vi "Mouse Down.vi"(8 "error in":errorcluster, 10 "Double Click":bool, 11 "Data in":T1={"Class"={"Ants"=refnum, "Layer"=refnum, "Templates"=refnum, "Icon"=refnum, "Glyph"=refnum, "Settings"=refnum, "Tools"=refnum, "History"=refnum}, "Ref"={"Add Layer"=refnum, "Remove Layer"=refnum, "Line Text"=[], "Body Text Spec"=refnum, "DNL_Font"=refnum, "glyph path str"=refnum, "templates path str"=refnum, "Arrow Up"=refnum, "Arrow Down"=refnum, "IE VI Ref"=refnum, "Glyphs tree"=refnum, "Templates tree"=refnum, "Layer Icon Text"=refnum, "Layer Template"=refnum, "Body Text"=refnum, "Search Templates"=refnum, "TextMarker"=refnum, "Tab Control"=refnum, "Search Glyphs"=refnum, "Line Color"=refnum, "DNL_Glyphs []"=refnum, "Fill Color"=refnum, "Tools"=refnum, "Icon"=refnum, "Preview"=refnum, "Ants"=refnum, "Terminals"=refnum, "menu reference"=refnum, "LayerNames"=[], "GlyphLoadAnimation"=refnum, "TemplateLoadAnimation"=refnum, "refreshGlyphs"=refnum, "refreshTemplates"=refnum}, "Support"={"AntsRect"={"left"=0, "top"=0, "right"=0, "bottom"=0}, "Mouse Move Coords"={"Horizontal"=0, "Vertical"=0}, "Mouse Down Coords"={"Horizontal"=0, "Vertical"=0}, "Temp Coord"={"Horizontal"=0, "Vertical"=0}, "Action"=enum."Default", "Edge Color"=4914962, "Fill Color"=16860, "Mouse Down?"=FALSE, "Draft Mode?"=FALSE, "Temp Icon"=bytes[3102], "CTRL Pressed"=FALSE, "Move Selection?"=FALSE, "AntsRect Orig"={"left"=0, "top"=0, "right"=0, "bottom"=0}, "Text"="", "TM Set?"=FALSE, "Mouse inside icon?"=FALSE, "Tool (old value)"=0, "Pencil Move Color"=0, "Swap Colors?"=FALSE, "Shift pressed?"=FALSE}}) -> (0 "error out":errorcluster, 3 "Data out":T1={"Class"={"Ants"=refnum, "Layer"=refnum, "Templates"=refnum, "Icon"=refnum, "Glyph"=refnum, "Settings"=refnum, "Tools"=refnum, "History"=refnum}, "Ref"={"Add Layer"=refnum, "Remove Layer"=refnum, "Line Text"=[], "Body Text Spec"=refnum, "DNL_Font"=refnum, "glyph path str"=refnum, "templates path str"=refnum, "Arrow Up"=refnum, "Arrow Down"=refnum, "IE VI Ref"=refnum, "Glyphs tree"=refnum, "Templates tree"=refnum, "Layer Icon Text"=refnum, "Layer Template"=refnum, "Body Text"=refnum, "Search Templates"=refnum, "TextMarker"=refnum, "Tab Control"=refnum, "Search Glyphs"=refnum, "Line Color"=refnum, "DNL_Glyphs []"=refnum, "Fill Color"=refnum, "Tools"=refnum, "Icon"=refnum, "Preview"=refnum, "Ants"=refnum, "Terminals"=refnum, "menu reference"=refnum, "LayerNames"=[], "GlyphLoadAnimation"=refnum, "TemplateLoadAnimation"=refnum, "refreshGlyphs"=refnum, "refreshTemplates"=refnum}, "Support"={"AntsRect"={"left"=0, "top"=0, "right"=0, "bottom"=0}, "Mouse Move Coords"={"Horizontal"=0, "Vertical"=0}, "Mouse Down Coords"={"Horizontal"=0, "Vertical"=0}, "Temp Coord"={"Horizontal"=0, "Vertical"=0}, "Action"=enum."Default", "Edge Color"=4914962, "Fill Color"=16860, "Mouse Down?"=FALSE, "Draft Mode?"=FALSE, "Temp Icon"=bytes[3102], "CTRL Pressed"=FALSE, "Move Selection?"=FALSE, "AntsRect Orig"={"left"=0, "top"=0, "right"=0, "bottom"=0}, "Text"="", "TM Set?"=FALSE, "Mouse inside icon?"=FALSE, "Tool (old value)"=0, "Pencil Move Color"=0, "Swap Colors?"=FALSE, "Shift pressed?"=FALSE}})   [LabVIEW 2020]
uses:
  Class/Ants/Ants.lvclass
  Class/FakedArray/FakedArray.lvclass
  vi.lib/LabVIEW Icon API/lv_icon/Classes/Icon/Icon.lvclass
  Class/Icon Library/Glyph.lvclass
  Class/Settings/Settings.lvclass
  Class/Tools/Tools Paint.lvclass
  History/History/History.lvclass
  vi.lib/LabVIEW Icon API/lv_icon/Controls/LayerType.ctl
  vi.lib/LabVIEW Icon API/lv_icon/Classes/Layer/Layer.lvclass
  History/History.lvlib
  <vilib>/Utility/miscctls.llb/LVPoint32TypeDef.ctl
  Controls/SupportClass_Action.ctl
  vi.lib/LabVIEW Icon API/lv_icon/Controls/IEColor.ctl
  Controls/Support Cluster.ctl
  lv_icon.lvlib
  Controls/References Cluster.ctl
  Controls/IE Classes.ctl
  Controls/Global Data.ctl
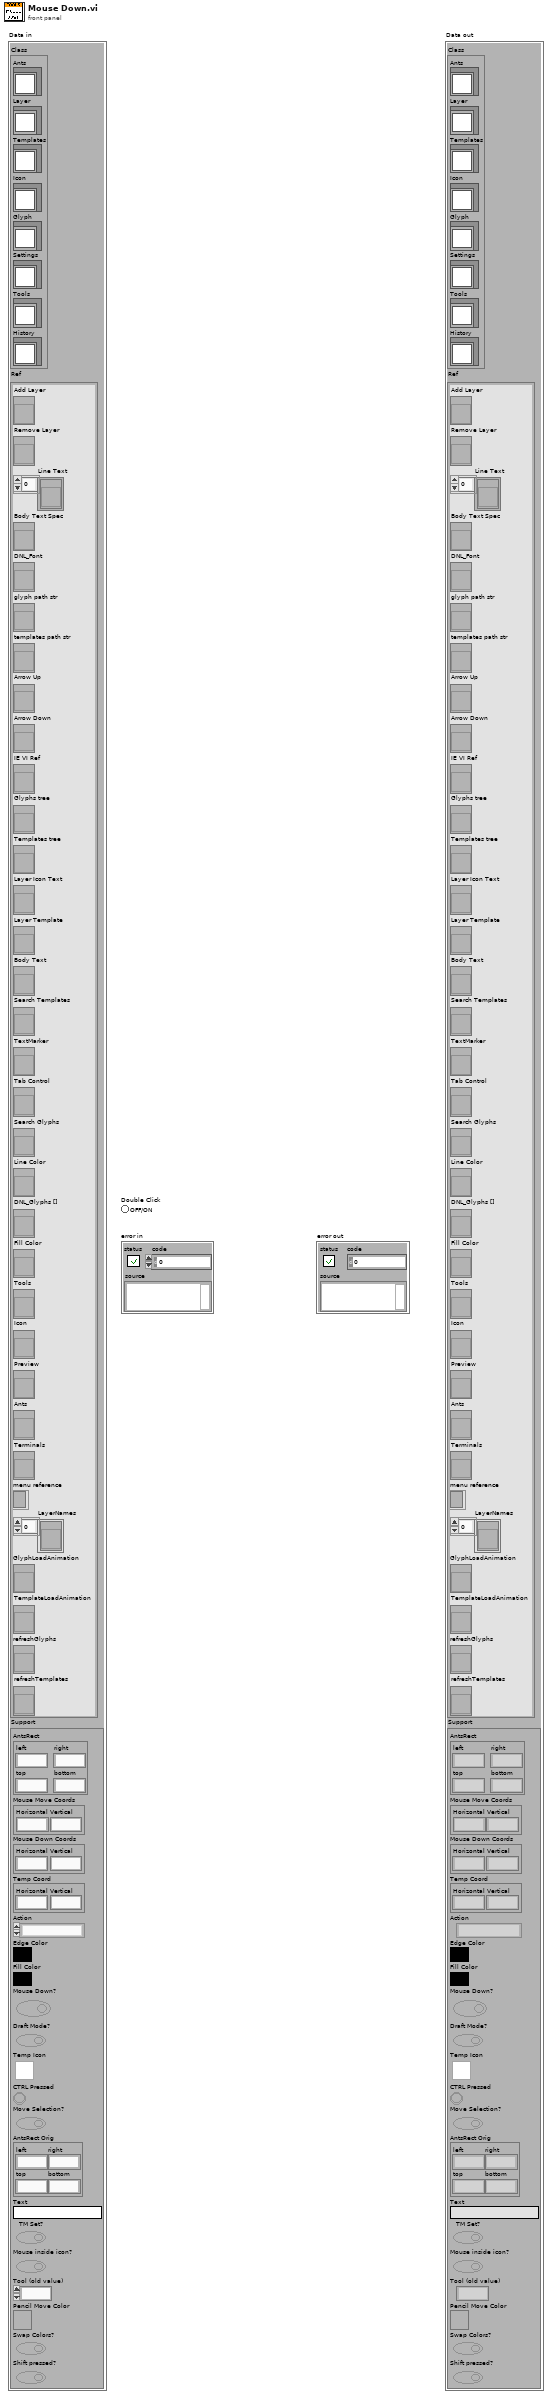
[diagram p1: front panel]
types:
  T1 = typedef "lv_icon.lvlib/Global Data.ctl" = cluster{"Class":T2, "Ref":T3, "Support":T4}
  T2 = typedef "lv_icon.lvlib/IE Classes.ctl" = cluster{"Ants":refnum<class "Ants.lvclass">, "Layer":refnum<class "FakedArray.lvclass">, "Templates":refnum<class "FakedArray.lvclass">, "Icon":refnum<class "Icon.lvclass">, "Glyph":refnum<class "Glyph.lvclass">, "Settings":refnum<class "Settings.lvclass">, "Tools":refnum<class "Tools Paint.lvclass">, "History":refnum<class "History.lvclass">}
  T3 = typedef "lv_icon.lvlib/References Cluster.ctl" = cluster{"Add Layer":refnum<vi>, "Remove Layer":refnum<vi>, "Line Text":refnum<vi>[], "Body Text Spec":refnum<vi>, "DNL_Font":refnum<vi>, "glyph path str":refnum<vi>, "templates path str":refnum<vi>, "Arrow Up":refnum<vi>, "Arrow Down":refnum<vi>, "IE VI Ref":refnum<vi>, "Glyphs tree":refnum<vi>, "Templates tree":refnum<vi>, "Layer Icon Text":refnum<vi>, "Layer Template":refnum<vi>, "Body Text":refnum<vi>, "Search Templates":refnum<vi>, "TextMarker":refnum<vi>, "Tab Control":refnum<vi>, "Search Glyphs":refnum<vi>, "Line Color":refnum<vi>, "DNL_Glyphs []":refnum<vi>, "Fill Color":refnum<vi>, "Tools":refnum<vi>, "Icon":refnum<vi>, "Preview":refnum<vi>, "Ants":refnum<vi>, "Terminals":refnum<vi>, "menu reference":refnum<k9>, "LayerNames":refnum<vi>[], "GlyphLoadAnimation":refnum<vi>, "TemplateLoadAnimation":refnum<vi>, "refreshGlyphs":refnum<vi>, "refreshTemplates":refnum<vi>}
  T4 = typedef "lv_icon.lvlib/Support Cluster.ctl" = cluster{"AntsRect":cluster{"left":i16, "top":i16, "right":i16, "bottom":i16}, "Mouse Move Coords":T5, "Mouse Down Coords":T5, "Temp Coord":T5, "Action":T6, "Edge Color":T7, "Fill Color":T7, "Mouse Down?":bool, "Draft Mode?":bool, "Temp Icon":picture, "CTRL Pressed":bool, "Move Selection?":bool, "AntsRect Orig":cluster{"left":i16, "top":i16, "right":i16, "bottom":i16}, "Text":string, "TM Set?":bool, "Mouse inside icon?":bool, "Tool (old value)":u32, "Pencil Move Color":u32, "Swap Colors?":bool, "Shift pressed?":bool}
  T5 = typedef "LVPoint32TypeDef.ctl" = cluster{"Horizontal":i32, "Vertical":i32}
  T6 = typedef "SupportClass_Action.ctl" = enum16{"Default", "Move Selection", "Glyph Library", "Tool"}
  T7 = typedef "IEColor.ctl" = u32
  T8 = typedef "LayerType.ctl" = enum16{"Graphic", "Text", "Tool", "Graphic Drop"}
  T9 = cluster{"left":i16, "top":i16, "right":i16, "bottom":i16}
  T10 = typedef "Tools.ctl" = enum32{"Pencil", "Line", "Dropper", "Fill", "Rectangle", "Filled Rectangle", "Ellipse", "Filled Ellipse", "Eraser", "Text", "Select", "Move"}
  T11 = typedef "lv_icon.lvlib/INI Data.ctl" = cluster{"Show Terminals?":bool, "Text":cluster{"Font":T12, "Alignment":T13, "Size":T14}, "3rd party Templates":cluster{"Store 3rd party Templates?":bool, "Folder Name":string}, "Merge user layers on commit":bool, "Body Text":T15, "Fill Color":T7, "Edge Color":T7, "Tab":u16, "Tool":T10, "Disable Layers?":bool}
  T12 = typedef "Font.ctl" = string
  T13 = typedef "Alignment.ctl" = u16
  T14 = typedef "Font Size.ctl" = u8
  T15 = typedef "BodyText.ctl" = cluster{"Line 1 text":string, "Line 2 text":string, "Line 3 text":string, "Line 4 text":string, "Line 1 color":u32, "Line 2 color":u32, "Line 3 color":u32, "Line 4 color":u32, "Body Text Spec":cluster{"Font":T12, "Alignment":T13, "Size":u8}, "Center text vertically":bool, "Capitalize Text":bool}
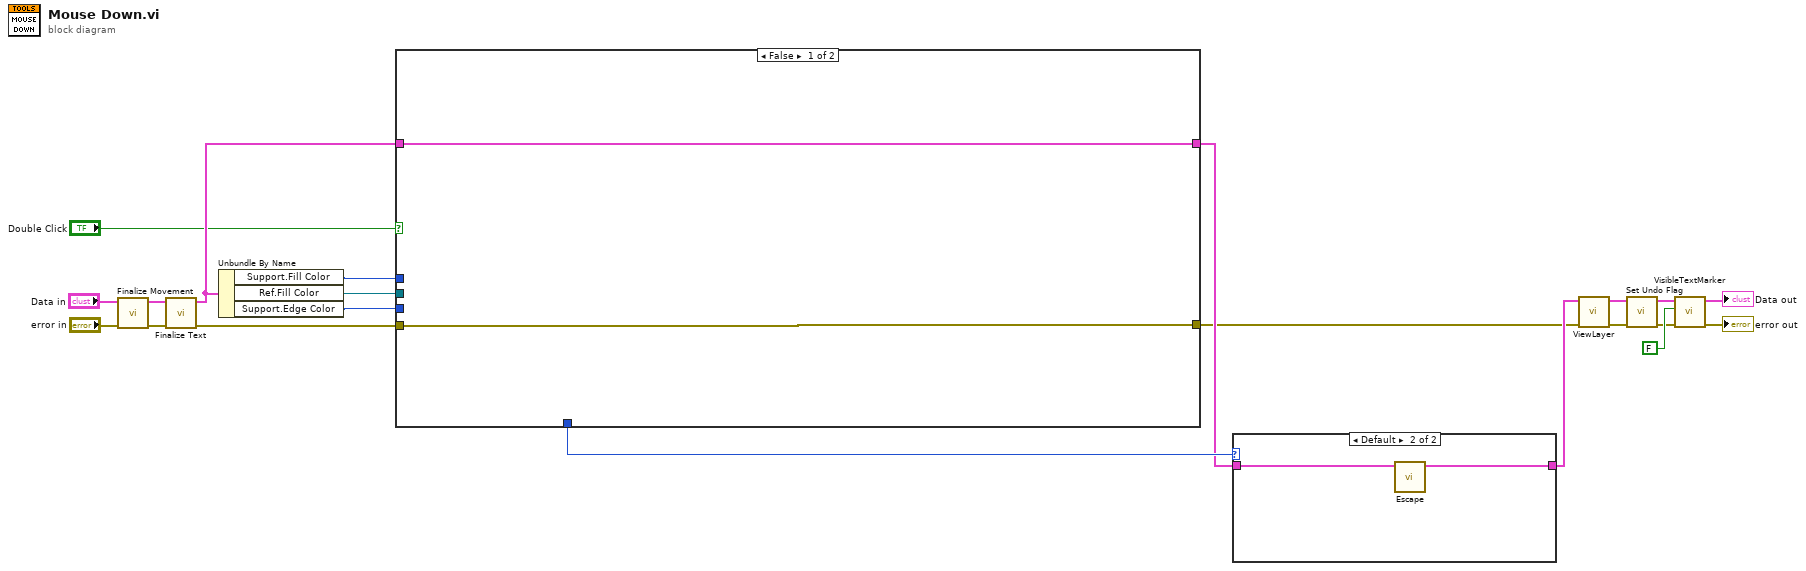
[diagram p0: block diagram]
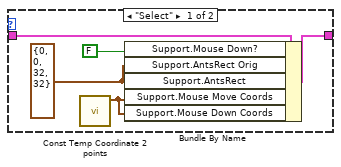
[diagram p2: hidden frame]
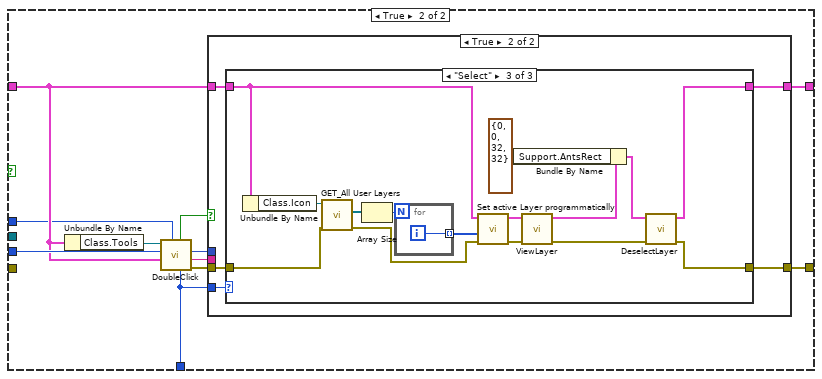
[diagram p3: hidden frame]
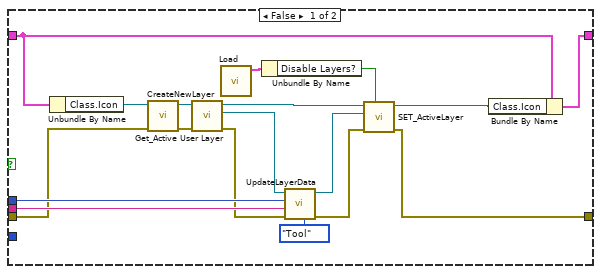
[diagram p4: hidden frame]
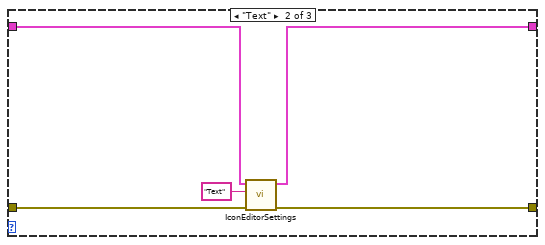
[diagram p6: hidden frame]
diagram:
  n1 = call "Finalize Movement.vi"("error in (no error)"="error in", "Data in"="Data in") -> ("error out"=w16:errorcluster, "Data out"=w14:T1)  [unwired: 1 in, 7 out]
  n2 = call "Finalize Text.vi"("error in (no error)"=w16, "Data in"=w14) -> ("error out"=w13:errorcluster, "Data out"=w2:T1)  [unwired: 8 out]
  n3 = Unbundle By Name(w2) -> ("Support.Fill Color"=w7:T7, "Ref.Fill Color"=w19:refnum<vi>, "Support.Edge Color"=w20:T7)
  n4 = case shown="False" "Double Click" {
    tunnel: w13 -> [w23 _]
    tunnel: w20 -> [_ w34]
    tunnel: [w23 w32] -> w8
    tunnel: [_ w28] -> w21
    tunnel: w19 -> [_ _]
    tunnel: w2 -> [w22 w26]
    tunnel: [w22 w25] -> w9
    tunnel: w7 -> [_ w24]
    frame False {
    }
    frame True {
      n5 = Unbundle By Name(w26) -> ("Class.Tools"=w27:refnum<class "Tools Paint.lvclass">)
      n6 = call "DoubleClick.vi"("Fill Color"=w24, "Data in"=w26, "Edge Color"=w34, "Tools Paint in"=w27) -> ("error out"=w33:errorcluster, "Name"=w30:string, "new picture"=w31:picture, "Active Tool"=w28:T10, "Invalid Picture?"=w29:bool)  [unwired: 1 in, 2 out]
      n7 = case shown="True" w29 {
        tunnel: w33 -> [w49 w56]
        tunnel: [w37 w55] -> w32
        tunnel: w31 -> [w52 _]
        tunnel: w30 -> [w51 _]
        tunnel: w28 -> [_ w57]
        tunnel: w26 -> [w38 w54]
        tunnel: [w50 w53] -> w25
        frame False {
          n8 = Unbundle By Name(w38) -> ("Class.Icon"=w40:refnum<class "Icon.lvclass">)
          n9 = call "CreateNewLayer.vi"("error in"=w49, "Icon.lvclass"=w40) -> ("error out"=w48:errorcluster, "Icon.lvclass out"=w47:refnum<class "Icon.lvclass">)  [unwired: 3 in, 5 out]
          n10 = call-dynamic "Get_Active User Layer.vi"("error in (no error)"=w48, "Icon in"=w47) -> ("error out"=w45:errorcluster, "Layer.lvclass"=w44:refnum<class "Layer.lvclass">, "Icon out"=w46:refnum<class "Icon.lvclass">)  [unwired: 7 out]
          n11 = call "Load.vi"() -> ("INI Data"=w36:T11)  [unwired: 3 in, 8 out]
          n12 = Unbundle By Name(w36) -> ("Disable Layers?"=w35:bool)
          n13 = call "UpdateLayerData.vi"("Type"=LayerType."Tool", "error in"=w45, "LayerName"=w51, "new picture"=w52, "Active Layer"=w44) -> ("error out"=w42:errorcluster, "Layer.lvclass out"=w43:refnum<class "Layer.lvclass">)  [unwired: 3 in, 2 out]
          n14 = call-dynamic "SET_ActiveLayer.vi"("Combine User Layers?"=w35, "error in (no error)"=w42, "Layer.lvclass"=w43, "Icon.lvclass in"=w46) -> ("error out"=w37:errorcluster, "Icon.lvclass out"=w39:refnum<class "Icon.lvclass">)  [unwired: 6 out]
          n15 = Bundle By Name(cluster=w38, "Class.Icon"=w39) -> (w50:T1)
        }
        frame True {
          n16 = case shown="\"Select\"" w57 {
            tunnel: w56 -> [w59 w64 w72]
            tunnel: [w59 w61 w65] -> w55
            tunnel: w54 -> [w58 w62 w71]
            tunnel: [w58 w60 w66] -> w53
            frame "Ellipse", Default {
            }
            frame "Text" {
              n17 = call "IconEditorSettings.vi"("error in (no error)"=w64, "Active Tag"="Text", "Data in"=w62) -> ("error out"=w61:errorcluster, "Data out"=w60:T1)  [unwired: 7 out]
            }
            frame "Select" {
              n18 = Unbundle By Name(w71) -> ("Class.Icon"=w70:refnum<class "Icon.lvclass">)
              n19 = call-dynamic "GET_All User Layers.vi"("error in (no error)"=w72, "Icon.lvclass in"=w70) -> ("error out"=w76:errorcluster, "User Layer"=w79:refnum<class "Layer.lvclass">[])  [unwired: 7 in, 1 out]
              n20 = Array Size(array=w79) -> (size(s)=w78:i32)
              n21 = for {
                N: w78 -> [_]
                tunnel: [w80] -> w77 mode=indexing
                i -> [w80]
              }
              n22 = call "Set active Layer programmatically.vi"("error in"=w76, "Active Layer []"=w77, "Data in"=w71) -> ("error out"=w73:errorcluster, "Data out"=w74:T1)  [unwired: 7 in]
              n23 = call "ViewLayer.vi"("error in (no error)"=w73, "Data in"=w74) -> ("error out"=w67:errorcluster, "Data out"=w69:T1)  [unwired: 2 in, 6 out]
              n24 = Bundle By Name(cluster=w69, "Support.AntsRect"=T9 {"left"=0, "top"=0, "right"=32, "bottom"=32}) -> (w68:T1)
              n25 = call "DeselectLayer.vi"("error in (no error)"=w67, "Data in"=w68) -> ("error out"=w65:errorcluster, "Data out"=w66:T1)  [unwired: 8 out]
            }
          }
        }
      }
    }
  }
  n26 = case shown="Default" w21 {
    tunnel: w9 -> [w83 w87]
    tunnel: [w82 w86] -> w12
    frame "Select" {
      w81 = T9 {"left"=0, "top"=0, "right"=32, "bottom"=32} ("Support.AntsRect Orig")
      n27 = call "Const Temp Coordinate 2 points.vi"() -> ("Const Temp Coordinate"=w84:T5)  [unwired: 11 out]
      n28 = Bundle By Name(cluster=w83, "Support.Mouse Down?"=FALSE ("Mouse Down?"), "Support.AntsRect Orig"=w81, "Support.AntsRect"=w81, "Support.Mouse Move Coords"=w84, "Support.Mouse Down Coords"=w84) -> (w82:T1)
    }
    frame Default {
      n29 = call "Escape.vi"("Data in"=w87) -> ("Data out"=w86:T1)  [unwired: 2 in, 8 out]
    }
  }
  n30 = call "ViewLayer.vi"("error in (no error)"=w8, "Data in"=w12) -> ("error out"=w17:errorcluster, "Data out"=w5:T1)  [unwired: 3 in, 5 out]
  n31 = call "Set Undo Flag.vi"("error in"=w17, "Data in"=w5) -> ("error out"=w6:errorcluster, "Data out"=w4:T1)  [unwired: 8 in]
  n32 = call "VisibleTextMarker.vi"("error in"=w6, "Visible"=FALSE, "Data in"=w4) -> ("error out"=→"error out":errorcluster, "Data out"=→"Data out":T1)  [unwired: 1 in, 6 out]
